vi "Single Count Test.vi"(0 "Start Measurement":bool, 1 "Сколько периодов копить":i32, 4 "Start-Stop1 Multyplex":T1, 5 "Window Length 1 (ns)":i32, 9 "Window Offset 1 (ns)":i32, 11 "Exposition Time (ms)":i64, 15 "Channel1 Threshold Voltage (mV)":i32 min=0 max=5000 step=10) -> (3 "Coincidence Count SS1":i64, 7 "Measurement index":i64, 10 "Total":i64, 12 "Exposition time (ms)":i64, 13 "Single Count Channel1":i64, 14 "Total":i64)   [LabVIEW 2012]
panel:
  in  "Stop Delay 1 (ns)":i16
  out "Single Count Channel4":i64
  out "Single Count Channel3":i64
  out "Single Count Channel2":i64
  out "Start OK":bool
  in  "Single Count Enable":T2
  in  "Channel4 Pulse Front":string
  in  "Channel4 Threshold Voltage (mV)":i32
  in  "Channel3 Pulse Front":string
  in  "Channel3 Threshold Voltage (mV)":i32
  in  "Channel2 Pulse Front":string
  in  "Channel2 Threshold Voltage (mV)":i32
  in  "Channel1 Pulse Front":string(combo)
  # "Start from 0\n0 -> Channel1\n1 -> Channel2"
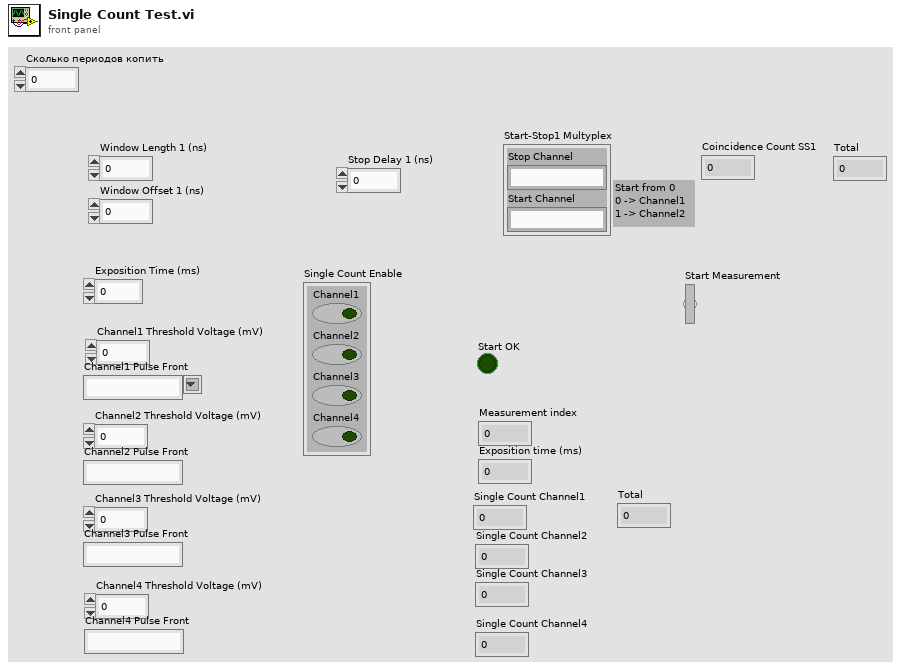
[diagram p1: front panel]
types:
  T1 = cluster{"Stop Channel":string, "Start Channel":string}
  T2 = cluster{"Channel1":bool, "Channel2":bool, "Channel3":bool, "Channel4":bool}
  T3 = cluster{"[0]":i64, "Channel1 Threshold Voltage (mV)":i32, "Channel1 Pulse Front":string, "Channel2 Threshold Voltage (mV)":i32, "Channel2 Pulse Front":string, "Channel3 Threshold Voltage (mV)":i32, "Channel3 Pulse Front ":string, "Channel4 Threshold Voltage (mV)":i32, "Channel4 Pulse Front ":string, "Single Count Enable":cluster{"Channel1":bool, "Channel2":bool, "Channel3":bool, "Channel4":bool}, "Single Count Max":i32, "Sum Count Enable":cluster{"Channel1":bool, "Channel2":bool, "Channel3":bool, "Channel4":bool}, "Sum Count Max":i32, "Start-Stop1 Multyplex":cluster{"Stop Channel":string, "Start Channel":string}, "Stop Delay 1 (ns)":i16, "Window Length 1 (ns)":i32, "Window Offset 1 (ns) ":i32, "Conditional Correlation 1":string, "Histogram Bin 1":string, "Histogram Start 1 (ns) ":i32, "Start-Stop2 Multyplex ":cluster{"Stop Channel":string, "Start Channel":string}, "Stop Delay 2 (ns)":i16, "Window Length 2 (ns) ":i32, "Window Offset 2 (ns) ":i32, "Conditional Correlation 2":string, "Histogram Bin 2":string, "Histogram Start 2 (ns)  ":i32, "Start-Stop3 Multyplex":cluster{"Stop Channel":string, "Start Channel":string}, "Stop Delay 3 (ns)":i16, "Window Length 3 (ns) ":i32, "Window Offset 3 (ns) ":i32, "Conditional Correlation 3":string, "Histogram Bin 3":string, "Histogram Start 3 (ns) ":i32, "Start-Stop4 Multyplex":cluster{"Stop Channel":string, "Start Channel":string}, "Stop Delay 4 (ns)":i16, "Window Length 4 (ns)  ":i32, "Window Offset 4 (ns) ":i32, "Conditional Correlation 4":string, "Histogram Bin 4":string, "Histogram Start 4 (ns)  ":i32, "Coincidence Count Enable":cluster{"Start-Stop1":bool, "Start-Stop2":bool, "Start-Stop3":bool, "Start-Stop4":bool}, "Coincidence Count Max":i32, "Coincidence Sum Enable":cluster{"Start-Stop1":bool, "Start-Stop2":bool, "Start-Stop3":bool, "Start-Stop4":bool}, "Coincidence Sum Max":i32, "Output Channel Enable":cluster{"Channel1":bool, "Channel2":bool, "Channel3":bool, "Channel4":bool}, "Output Channel Inversion":cluster{"Channel1":bool, "Channel2":bool, "Channel3":bool, "Channel4":bool, "Output":bool}}
  T4 = cluster{"Going":bool, "Iinterrupted":bool, "Timer stop":bool, "Single count stop Ch1":bool, "Single count stop Ch2":bool, "Single count stop Ch3":bool, "Single count stop Ch4":bool, "Sum count stop":bool, "Coincidence count stop SS1":bool, "Coincidence count stop SS2":bool, "Coincidence count stop SS3":bool, "Coincidence count stop SS4":bool, "Coincidence sum count stop":bool, "Reserved":bool, "Correlator is not initialised":bool, "Internal error":bool}
  T5 = cluster{"Measurement index":i64, "Exposition time (ms)":i64, "Single Count Channel1":i64, "Single Count Channel2":i64, "Single Count Channel3":i64, "Single Count Channel4":i64, "Sum Single Count":i64, "Coincidence Count SS1":i64, "Coincidence Count SS2":i64, "Coincidence Count SS4":i64, "Coincidence Count SS5":i64, "Sum Coincidence Count":i64}
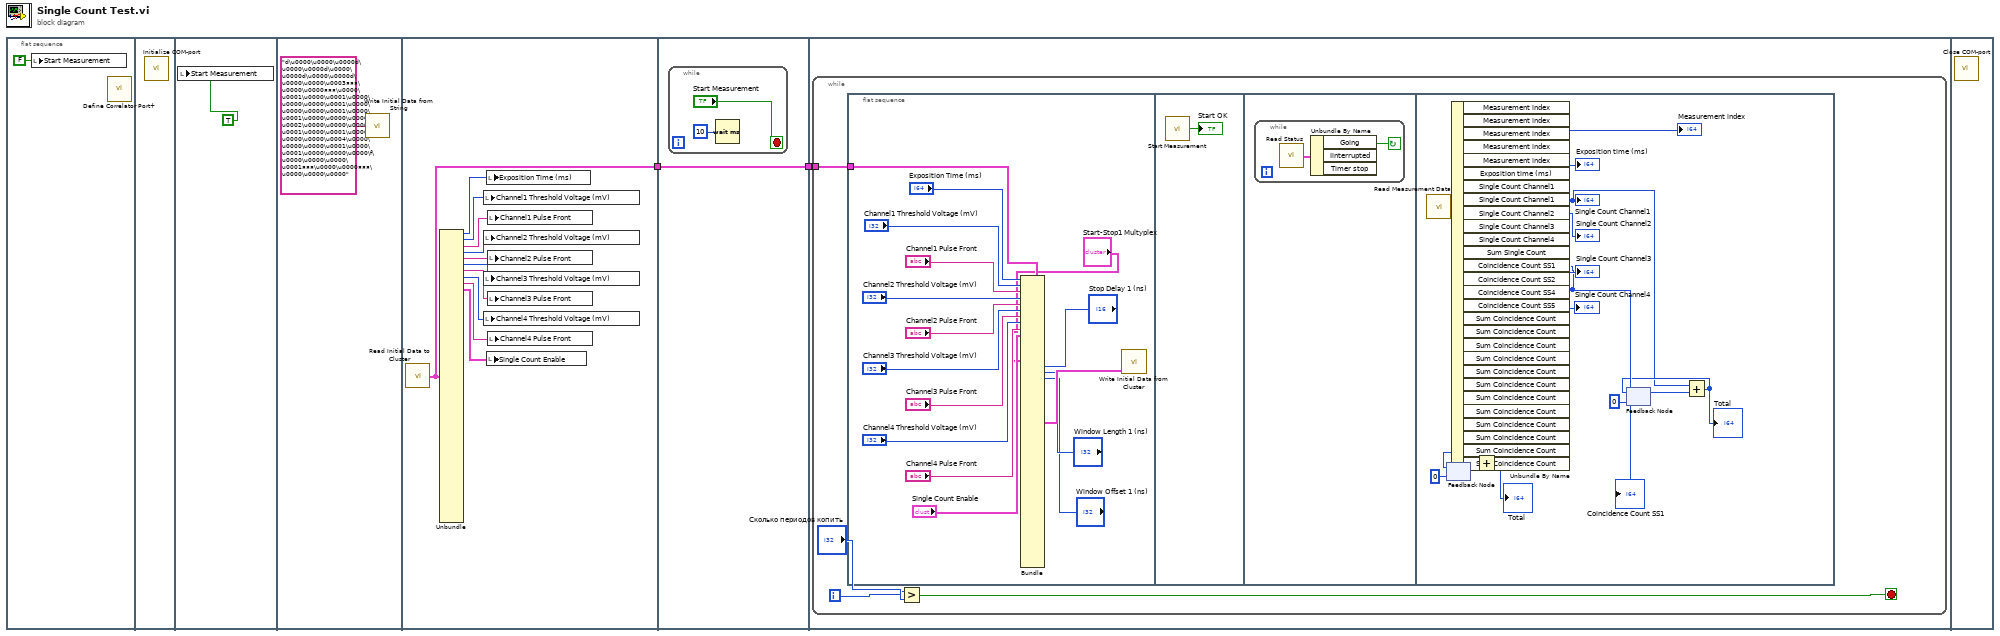
[diagram p0: block diagram]
diagram:
  n1 = flat-sequence {
    tunnel: [w16] -> w2
    tunnel: w2 -> [w17]
    tunnel: [w17] -> w1
    tunnel: w1 -> [w20]
    frame #0 {
      n2 = local write "Start Measurement"(FALSE ("Start Measurement")) -> ()
      n3 = call "Define Correlator Port+.vi"() -> ()  [unwired: 3 in]
    }
    frame #1 {
      n4 = call "Initialize COM-port.vi"() -> ()  [unwired: 4 in]
    }
    frame #2 {
      n5 = local write "Start Measurement"(TRUE ("Start Measurement")) -> ()
    }
    frame #3 {
      n6 = call "Write Initial Data from String.vi"("Data"="d\u0000\u0000\u0000d\u0000\u0000d\u0000\u0000d\u0000\u0000d\u0000\u0000\u0003яяя\u0000\u0000яяя\u0000\u0001\u0000\u0001\u0000\u0000\u0000\u0001\u0000\u0000\u0000\u0001\u0000\u0001\u0000\u0000\u0000\u0002\u0000\u0000\u0000\u0001\u0000\u0001\u0000\u0000\u0000\u0004\u0000\u0000\u0000\u0001\u0000\u0001\u0000\u0000\u0000\f\u0000\u0000\u0000\u0001яяя\u0000\u0000яяя\u0000\u0000\u0000") -> ()  [unwired: 1 out]
    }
    frame #4 {
      n7 = call "Read Initial Data to Cluster.vi"() -> ("Correlator Initial Data 2"=w16:T3)  [unwired: 2 in]
      n8 = Unbundle(w16) -> ("[0]"=w15:i64, "Channel1 Threshold Voltage (mV)"=w14:i32, "Channel1 Pulse Front"=w13:string, "Channel2 Threshold Voltage (mV)"=w12:i32, "Channel2 Pulse Front"=w11:string, "Channel3 Threshold Voltage (mV)"=w10:i32, "Channel3 Pulse Front"=w9:string, "Channel4 Threshold Voltage (mV)"=w8:i32, "Channel4 Pulse Front"=w7:string, "Single Count Enable"=w6:T2)  [unwired: 37 out]
      n9 = local write "Channel1 Threshold Voltage (mV)"(w14) -> ()
      n10 = local write "Channel2 Threshold Voltage (mV)"(w12) -> ()
      n11 = local write "Channel3 Threshold Voltage (mV)"(w10) -> ()
      n12 = local write "Channel4 Threshold Voltage (mV)"(w8) -> ()
      n13 = local write "Exposition Time (ms)"(w15) -> ()
      n14 = local write "Single Count Enable"(w6) -> ()
      n15 = local write "Channel1 Pulse Front"(w13) -> ()
      n16 = local write "Channel2 Pulse Front"(w11) -> ()
      n17 = local write "Channel3 Pulse Front"(w9) -> ()
      n18 = local write "Channel4 Pulse Front"(w7) -> ()
    }
    frame #5 {
      n19 = while {
        stop <- "Start Measurement" stop-if-true
        n20 = Wait (ms)(milliseconds to wait=u32 10) -> ()  [unwired: 1 out]
      }
    }
    frame #6 {
      n21 = while {
        tunnel: w20 -> [w24]
        i -> [w22]
        stop <- w21 stop-if-true
        n22 = flat-sequence {
          tunnel: w24 -> [w32]
          frame #0 {
            n23 = Bundle(cluster=w32, "[0]"="Exposition Time (ms)", "Channel1 Threshold Voltage (mV)"="Channel1 Threshold Voltage (mV)", "Channel1 Pulse Front"="Channel1 Pulse Front", "Channel2 Threshold Voltage (mV)"="Channel2 Threshold Voltage (mV)", "Channel2 Pulse Front"="Channel2 Pulse Front", "Channel3 Threshold Voltage (mV)"="Channel3 Threshold Voltage (mV)", "Channel3 Pulse Front"="Channel3 Pulse Front", "Channel4 Threshold Voltage (mV)"="Channel4 Threshold Voltage (mV)", "Channel4 Pulse Front"="Channel4 Pulse Front", "Single Count Enable"="Single Count Enable", "Start-Stop1 Multyplex"="Start-Stop1 Multyplex", "Stop Delay 1 (ns)"="Stop Delay 1 (ns)", "Window Length 1 (ns)"="Window Length 1 (ns)", "Window Offset 1 (ns)"="Window Offset 1 (ns)") -> (w40:T3)  [unwired: 33 in]
            n24 = call "Write Initial Data from Cluster.vi"("Correlator Initial Data"=w40) -> ()  [unwired: 2 in, 1 out]
          }
          frame #1 {
            n25 = call "Start Measurement.vi"() -> ("Start OK"=→"Start OK":bool)  [unwired: 2 in]
          }
          frame #2 {
            n26 = while {
              stop <- w42 continue-if-true
              n27 = call "Read Status.vi"() -> ("Status Data"=w43:T4)  [unwired: 2 in]
              n28 = Unbundle By Name(w43) -> ("Going"=w42:bool)  [unwired: 2 out]
            }
          }
          frame #3 {
            n29 = call "Read Measurement Data.vi"() -> ("Measurement Data"=w57:T5)  [unwired: 3 in]
            n30 = feedback #1(i64 0) -> (w52:i64)
            n31 = Unbundle By Name(w57) -> ("Measurement index"=→"Measurement index":i64, "Exposition time (ms)"=→"Exposition time (ms)":i64, "Single Count Channel1"=w47:i64, "Single Count Channel2"=→"Single Count Channel2":i64, "Single Count Channel3"=→"Single Count Channel3":i64, "Single Count Channel4"=→"Single Count Channel4":i64, "Coincidence Count SS1"=w50:i64)  [unwired: 21 out]
            "Single Count Channel1" <- w47
            "Coincidence Count SS1" <- w50
            n32 = Add(x=w50, y=w52) -> (x+y=w51:i64)
            "Total" <- w51
            n33 = feedback-in #1(w51) -> ()
            n34 = feedback #2(i64 0) -> (w49:i64)
            n35 = Add(x=w47, y=w49) -> (x+y=w48:i64)
            "Total" <- w48
            n36 = feedback-in #2(w48) -> ()
          }
        }
        n37 = Greater?(x=w22, y="Сколько периодов копить") -> (0:w21:bool)
      }
    }
    frame #7 {
      n38 = call "Close COM-port.vi"() -> ()  [unwired: 4 in]
    }
  }
